vi "GetErrorBehavior.vi"(8 "error in (no error)":errorcluster, 11 "SMO in":refnum<class "SMO.lvclass">) -> (0 "error out":errorcluster, 2 "Shutdown on Unhandled Error":bool, 3 "SMO out":refnum<class "SMO.lvclass">)   [LabVIEW 2021, in "smo.lvlib" / "SMO.lvclass"]
uses:
  SMO.lvclass
  Support/Attribute.ErrorHandling/Attribute.ErrorHandling.lvclass
  SMO.lvclass/SMO.ctl
  Support/Attribute.ErrorHandling/Attribute.ErrorHandling.lvclass/Attribute.ErrorHandling.ctl
  ReftoDVR--SMO.vi
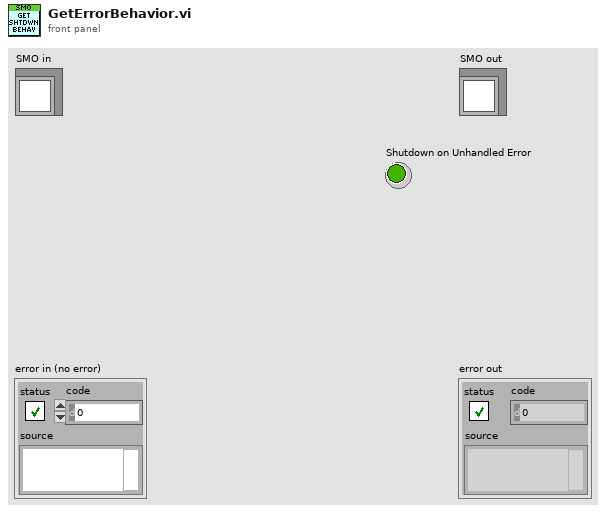
[diagram p1: front panel]
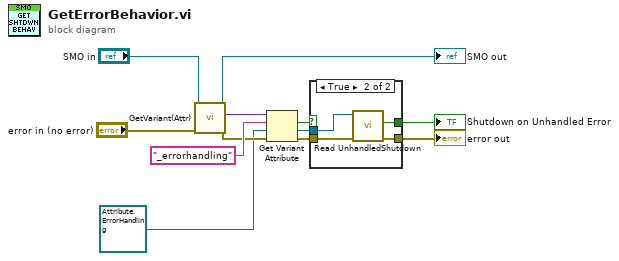
[diagram p0: block diagram]
diagram:
  n1 = call "GetVariant(Attr).vi"("error in (no error)"="error in (no error)", "SMO in"="SMO in") -> ("error out"=w10:errorcluster, "[Attributes]"=w12:variant, "SMO out"=→"SMO out":refnum<class "SMO.lvclass">)  [unwired: 7 in]
  n2 = Get Variant Attribute(Variant=w12, name="_errorhandling", default value (empty Variant)=refnum<class "Attribute.ErrorHandling.lvclass"> refnum ("Attribute.ErrorHandling.lvclass"), error in=w10) -> (found=w1:bool, value=w5:refnum<class "Attribute.ErrorHandling.lvclass">, error out=w4:errorcluster)  [unwired: 1 out]
  n3 = case shown="True" w1 {
    tunnel: w5 -> [_ w17]
    tunnel: w4 -> [w13 w16]
    tunnel: [w13 w15] -> w3
    tunnel: [_ w14] -> w2
    frame False {
    }
    frame True {
      n4 = call "Read UnhandledShutdown.vi"("error in (no error)"=w16, "Attribute.StartupBehavior in"=w17) -> ("error out"=w15:errorcluster, "Shutdown on Unhandled Error"=w14:bool)  [unwired: 7 in, 1 out]
    }
  }
  "error out" <- w3
  "Shutdown on Unhandled Error" <- w2
